vi "Agilent VNA Set Measurement Format.vi"(6 "Channel":i32=1 min=1 max=99 step=1 format="%#_2f", 7 "Agilent VNA":T1, 8 "error in (no error)":errorcluster, 10 "Measurement Format (Log Mag)":T2, 11 "VISA Resource Name":refnum<visa-resource-name>) -> (0 "error out":errorcluster, 3 "dup VISA Resource Name":refnum<visa-resource-name>)   [LabVIEW 2011]
doc: "This VI for the HP8753B is used to set the meausurement format."
uses:
  Agilent VNA Measurement Format.ctl
  TypeDefs/Agilent VNA Instrument Info.ctl
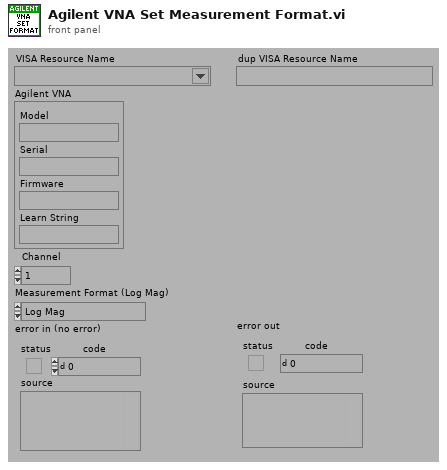
[diagram p1: front panel]
types:
  T1 = typedef "Agilent VNA Instrument Info.ctl" = cluster{"Model":string, "Serial":string, "Firmware":string, "Learn String":string}
  T2 = typedef "Agilent VNA Measurement Format.ctl" = enum32{"Log Mag", "Phase", "Delay", "Smith (R+jX)", "Polar (Re/Im)", "Linear Mag", "SWR", "Real", "Imaginary", "Smith (Lin/Phase)", "Smith (Log/Phase)", "Smith (Real/Imag)", "Smith (G+jB)", "Polar (Lin)", "Polar (Log)", "Expanded Phase", "Positive Phase"}
  T3 = typedef "SP Measurement Format.ctl" = enum32{"Log Mag", "Phase", "Delay", "Smith (R+jX)", "Polar (Re/Im)", "Linear Mag", "SWR", "Real", "Imaginary", "Smith (Lin/Phase)", "Smith (Log/Phase)", "Smith (Real/Imag)", "Smith (G+jB)", "Polar (Lin/Phase)", "Polar (Log/Phase)", "Expanded Phase", "Positive Phase", "Inverted Smith", "Unwrapped Phase", "Power Out", "Power In", "Linear Mag/Phase", "Log Mag/Phase", "Real/Imaginary"}
  T4 = typedef "Agilent VNA Model.ctl" = enum16{"Not Supported", "8510X", "8719X", "8720X", "8722X", "8753X", "ENA", "PNA", "Field Fox"}
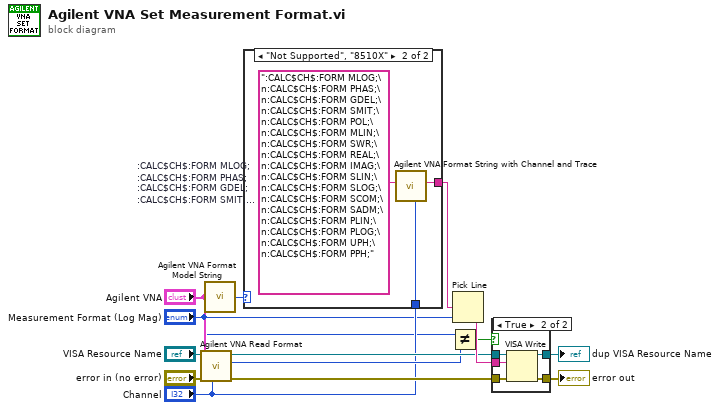
[diagram p0: block diagram]
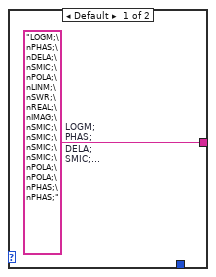
[diagram p2: hidden frame]
diagram:
  n1 = call "Agilent VNA Read Format.vi"("Channel"="Channel", "Agilent VNA"="Agilent VNA", "error in (no error)"="error in (no error)", "VISA Resource Name"="VISA Resource Name") -> ("error out"=w8:errorcluster, "Display Format"=w6:T3, "dup VISA Resource Name"=w7:refnum<visa-resource-name>)  [unwired: 5 in]
  n2 = call "Agilent VNA Format Model String.vi"("Model"="Agilent VNA") -> ("Model"=w4:T4)
  n3 = case shown="\"E5070B\", \"E5071B\"" w4 {
    tunnel: [w15 w17] -> w12
    tunnel: "Channel" -> [_ w16]
    frame Default {
      w15 = "LOGM;\nPHAS;\nDELA;\nSMIC;\nPOLA;\nLINM;\nSWR;\nREAL;\nIMAG;\nSMIC;\nSMIC;\nSMIC;\nSMIC;\nPOLA;\nPOLA;\nPHAS;\nPHAS;"  # LOGM; PHAS; DELA; SMIC; POLA; LINM; SWR; REAL; IMAG; SMIC; SMIC; SMIC; SMIC; POLA; POLA; PHAS; PHAS;
    }
    frame "Not Supported", "8510X" {
      w18 = ":CALC$CH$:FORM MLOG;\n:CALC$CH$:FORM PHAS;\n:CALC$CH$:FORM GDEL;\n:CALC$CH$:FORM SMIT;\n:CALC$CH$:FORM POL;\n:CALC$CH$:FORM MLIN;\n:CALC$CH$:FORM SWR;\n:CALC$CH$:FORM REAL;\n:CALC$CH$:FORM IMAG;\n:CALC$CH$:FORM SLIN;\n:CALC$CH$:FORM SLOG;\n:CALC$CH$:FORM SCOM;\n:CALC$CH$:FORM SADM;\n:CALC$CH$:FORM PLIN;\n:CALC$CH$:FORM PLOG;\n:CALC$CH$:FORM UPH;\n:CALC$CH$:FORM PPH;"  # :CALC$CH$:FORM MLOG; :CALC$CH$:FORM PHAS; :CALC$CH$:FORM GDEL; :CALC$CH$:FORM SMIT; :CALC$CH$:FORM POL; :CALC$CH$:FORM MLIN; :CALC$CH$:FORM SWR; :CALC$CH$:FORM REAL; :CALC$CH$:FORM IMAG; :CALC$CH$:FORM SLIN; :CALC$CH$:FORM SLOG; :CALC$CH$:FORM SCOM; :CALC$CH$:FORM SADM; :CALC$CH$:FORM PLIN; :CALC$CH$:FORM PLOG; :CALC$CH$:FORM UPH; :CALC$CH$:FORM PPH;
      n4 = call "Agilent VNA Format String with Channel and Trace.vi"("Trace"=w16, "String"=w18) -> ("String Out"=w17:string)  [unwired: 7 in]
    }
  }
  n5 = Not Equal?(x="Measurement Format (Log Mag)", y=w6) -> (x != y?=w5:bool)
  n6 = Pick Line(multi-line string=w12, line index="Measurement Format (Log Mag)") -> (output string=w11:string)  [unwired: 1 in]
  n7 = case shown="True" w5 {
    tunnel: [w20 w25] -> w14
    tunnel: [w19 w24] -> w13
    tunnel: w11 -> [_ w23]
    tunnel: w8 -> [w19 w22]
    tunnel: w7 -> [w20 w21]
    frame False {
    }
    frame True {
      n8 = VISA Write(VISA resource name=w21, write buffer=w23, error in (no error)=w22) -> (VISA resource name out=w25:refnum<visa-resource-name>, error out=w24:errorcluster)  [unwired: 1 out]
    }
  }
  "dup VISA Resource Name" <- w14
  "error out" <- w13
